vi "GF_PusleChannel1ms.vi"(1 "error in":errorcluster, 2 "DAQmx Global Channel":refnum<k21>="USB_TurnOffBProbeRelay_P0_4") -> (0 "error out":errorcluster)   [LabVIEW 2016]
uses:
  <vilib>/DAQmx/write.llb/DAQmx Write (Digital Bool 1Line 1Point).vi
  <vilib>/DAQmx/miscellaneous.llb/DAQmx Fill In Error Info.vi
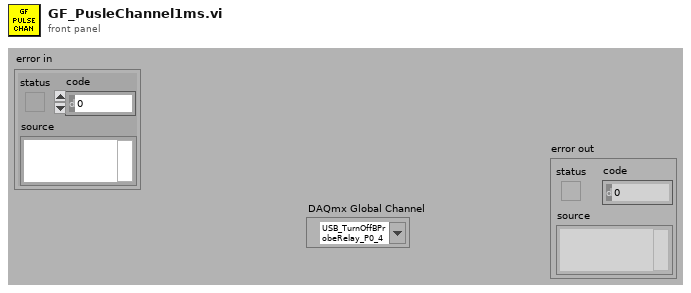
[diagram p1: front panel]
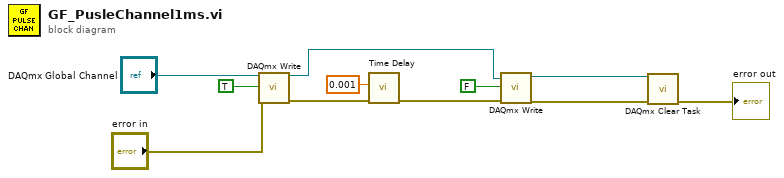
[diagram p0: block diagram]
diagram:
  n1 = call-poly <vilib>:"DAQmx Write.vi"("task/channels in"="DAQmx Global Channel", "data"=TRUE, "error in"="error in") -> ("task out"=w7:refnum<k21>, "error out"=w9:errorcluster)  [unwired: 10 in, 1 out]
  n2 = call "Time Delay"("error in (no error)"=w9, "Delay Time (s)"=0.001) -> ("error out"=w6:errorcluster)  [unwired: 9 in]
  n3 = call-poly <vilib>:"DAQmx Write.vi"("task/channels in"=w7, "data"=FALSE, "error in"=w6) -> ("task out"=w5:refnum<k21>, "error out"=w4:errorcluster)  [unwired: 10 in, 1 out]
  n4 = call <vilib>:"DAQmx Clear Task.vi"("task in"=w5, "error in"=w4) -> ("error out"=→"error out":errorcluster)  [unwired: 13 in]
